vi "Start_rate.vi"(0 "TCP connection ID":refnum<k5>, 5 "UDP connection ID":refnum<k16>, 7 "IP address in":u32, 12 "error in":errorcluster) -> (4 "TCP connection ID out":refnum<k5>, 6 "UDP connection ID out":refnum<k16>, 8 "IP address out":u32, 10 "timeout ms (25000)":i32=1000, 14 "error out":errorcluster)   [LabVIEW 2017]
panel:
  out "String 5":string
  out "String 4":string
  out "String 3":string
  out "String 2":string
  out "String 1":string
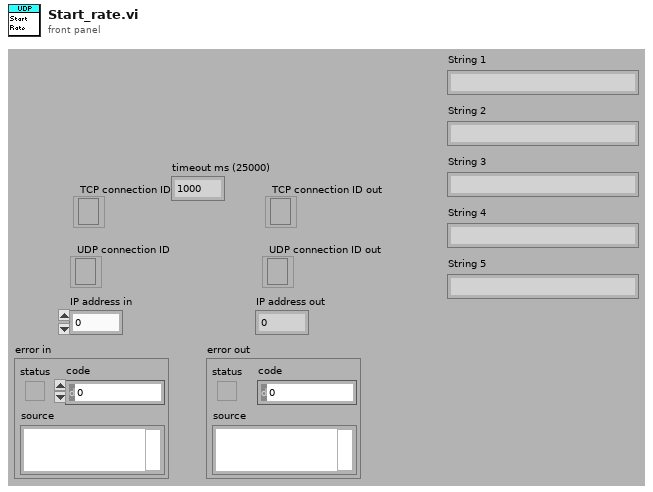
[diagram p1: front panel]
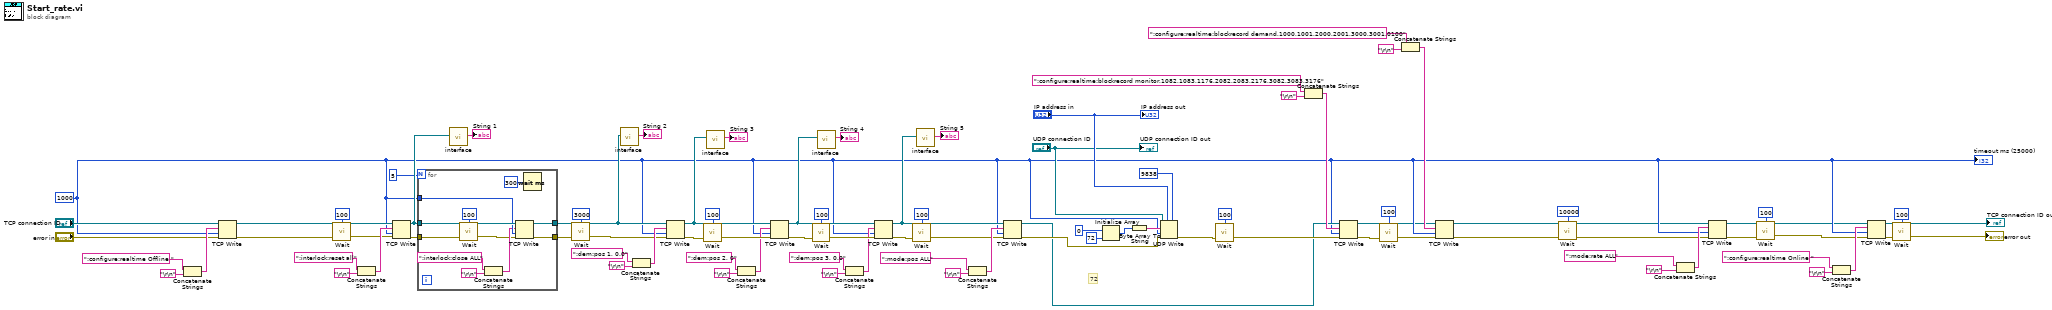
[diagram p0: block diagram]
diagram:
  w12 = 1000 ("timeout ms (25000)")
  # "72"
  n1 = Concatenate Strings(":configure:realtime Offline " ("ACL Command"), "\r\n") -> (w19:string)
  n2 = TCP Write(connection ID="TCP connection ID", data in=w19, error in (no error)="error in", 9:w12) -> (connection ID out=w16:refnum<k5>, error out=w15:errorcluster)  [unwired: 1 out]
  n3 = call "Wait.vi"("Wartezeit in ms"=u32 100, "error in (no error)"=w15) -> ("error out"=w35:errorcluster)  [unwired: 3 in]
  n4 = Concatenate Strings(":interlock:reset all" ("ACL Command"), "\r\n") -> (w38:string)
  n5 = TCP Write(connection ID=w16, data in=w38, error in (no error)=w35, 9:w12) -> (connection ID out=w60:refnum<k5>, error out=w37:errorcluster)  [unwired: 1 out]
  n6 = for {
    N: 5 -> [_]
    tunnel: w60 -> [w100]
    tunnel: [w99] -> w54
    tunnel: [w98] -> w50
    tunnel: w12 -> [w97]
    tunnel: w37 -> [w93]
    n7 = call "Wait.vi"("Wartezeit in ms"=u32 100, "error in (no error)"=w93) -> ("error out"=w92:errorcluster)  [unwired: 3 in]
    n8 = Concatenate Strings(":interlock:close ALL" ("ACL Command"), "\r\n") -> (w94:string)
    n9 = TCP Write(connection ID=w100, data in=w94, error in (no error)=w92, 9:w97) -> (connection ID out=w99:refnum<k5>, error out=w98:errorcluster)  [unwired: 1 out]
    n10 = Wait (ms)(milliseconds to wait=u32 300) -> ()  [unwired: 1 out]
  }
  n11 = call "interface.vi"("TCP Network Connection Refnum"=w60) -> ("String"=→"String 1":string)  [unwired: 8 in, 2 out]
  n12 = call "Wait.vi"("Wartezeit in ms"=u32 3000, "error in (no error)"=w50) -> ("error out"=w61:errorcluster)  [unwired: 3 in]
  n13 = call "interface.vi"("TCP Network Connection Refnum"=w54) -> ("String"=→"String 2":string)  [unwired: 8 in, 2 out]
  n14 = Concatenate Strings(":dem:pos 1, 0.0" ("ACL Command"), "\r\n") -> (w62:string)
  n15 = TCP Write(connection ID=w54, data in=w62, error in (no error)=w61, 9:w12) -> (connection ID out=w53:refnum<k5>, error out=w78:errorcluster)  [unwired: 1 out]
  n16 = call "Wait.vi"("Wartezeit in ms"=u32 100, "error in (no error)"=w78) -> ("error out"=w80:errorcluster)  [unwired: 3 in]
  n17 = call "interface.vi"("TCP Network Connection Refnum"=w53) -> ("String"=→"String 3":string)  [unwired: 8 in, 2 out]
  n18 = Concatenate Strings(":dem:pos 2, 0" ("ACL Command"), "\r\n") -> (w63:string)
  n19 = TCP Write(connection ID=w53, data in=w63, error in (no error)=w80, 9:w12) -> (connection ID out=w52:refnum<k5>, error out=w75:errorcluster)  [unwired: 1 out]
  n20 = call "Wait.vi"("Wartezeit in ms"=u32 100, "error in (no error)"=w75) -> ("error out"=w76:errorcluster)  [unwired: 3 in]
  n21 = call "interface.vi"("TCP Network Connection Refnum"=w52) -> ("String"=→"String 4":string)  [unwired: 8 in, 2 out]
  n22 = Concatenate Strings(":dem:pos 3, 0.0" ("ACL Command"), "\r\n") -> (w64:string)
  n23 = TCP Write(connection ID=w52, data in=w64, error in (no error)=w76, 9:w12) -> (connection ID out=w32:refnum<k5>, error out=w73:errorcluster)  [unwired: 1 out]
  n24 = call "Wait.vi"("Wartezeit in ms"=u32 100, "error in (no error)"=w73) -> ("error out"=w33:errorcluster)  [unwired: 3 in]
  n25 = call "interface.vi"("TCP Network Connection Refnum"=w32) -> ("String"=→"String 5":string)  [unwired: 8 in, 2 out]
  n26 = Concatenate Strings(":mode:pos ALL" ("ACL Command"), "\r\n") -> (w65:string)
  n27 = TCP Write(connection ID=w32, data in=w65, error in (no error)=w33, 9:w12) -> (connection ID out=w29:refnum<k5>, error out=w30:errorcluster)  [unwired: 1 out]
  n28 = Initialize Array(u8 0, 72 ("dimension size")) -> (w84:u8[])
  n29 = Byte Array To String(unsigned byte array=w84) -> (string=w83:string)
  n30 = UDP Write(address="IP address in", port or service name=u16 9838 ("Remote Port"), connection ID="UDP connection ID", data in=w83, 8:w30, 9:w12) -> (error out=w81:errorcluster)  [unwired: 1 out]
  n31 = call "Wait.vi"("Wartezeit in ms"=u32 100, "error in (no error)"=w81) -> ("error out"=w43:errorcluster)  [unwired: 3 in]
  n32 = Concatenate Strings(":configure:realtime:blockrecord monitor,1082,1083,1176,2082,2083,2176,3082,3083,3176" ("ACL Command"), "\r\n") -> (w48:string)
  n33 = TCP Write(connection ID=w29, data in=w48, error in (no error)=w43, 9:w12) -> (connection ID out=w1:refnum<k5>, error out=w3:errorcluster)  [unwired: 1 out]
  n34 = call "Wait.vi"("Wartezeit in ms"=u32 100, "error in (no error)"=w3) -> ("error out"=w2:errorcluster)  [unwired: 3 in]
  n35 = Concatenate Strings(":configure:realtime:blockrecord demand,1000,1001,2000,2001,3000,3001,0100" ("string"), "\r\n") -> (w45:string)
  n36 = TCP Write(connection ID=w1, data in=w45, error in (no error)=w2, 9:w12) -> (connection ID out=w6:refnum<k5>, error out=w5:errorcluster)  [unwired: 1 out]
  n37 = call "Wait.vi"("Wartezeit in ms"=u32 10000, "error in (no error)"=w5) -> ("error out"=w7:errorcluster)  [unwired: 3 in]
  n38 = Concatenate Strings(":mode:rate ALL" ("ACL Command"), "\r\n") -> (w13:string)
  n39 = TCP Write(connection ID=w6, data in=w13, error in (no error)=w7, 9:w12) -> (connection ID out=w10:refnum<k5>, error out=w11:errorcluster)  [unwired: 1 out]
  n40 = call "Wait.vi"("Wartezeit in ms"=u32 100, "error in (no error)"=w11) -> ("error out"=w23:errorcluster)  [unwired: 3 in]
  n41 = Concatenate Strings(":configure:realtime Online " ("ACL Command"), "\r\n") -> (w25:string)
  n42 = TCP Write(connection ID=w10, data in=w25, error in (no error)=w23, 9:w12) -> (connection ID out=→"TCP connection ID out":refnum<k5>, error out=w28:errorcluster)  [unwired: 1 out]
  n43 = call "Wait.vi"("Wartezeit in ms"=u32 100, "error in (no error)"=w28) -> ("error out"=→"error out":errorcluster)  [unwired: 3 in]
  "UDP connection ID out" <- "UDP connection ID"
  "IP address out" <- "IP address in"
  "timeout ms (25000)" <- w12
